vi "Read from File.vi"(7 "Section Name":string, 8 "error in (no error)":errorcluster, 10 "INI Ref":T1, 11 "Window Action in":refnum<class "Window Action.lvclass">) -> (0 "error out":errorcluster, 2 "INI Ref out":T1, 3 "Window Action out":refnum<class "Window Action.lvclass">)   [LabVIEW 2020, in "MacroAssert.lvlib" / "Window Action.lvclass"]
doc: "Reads associated parameters from the file identified by <B>INI Ref</B>."
uses:
  Window Action.lvclass
  <vilib>/Utility/config.llb/Config Data RefNum.ctl
  Window Action Type.ctl
  <vilib>/Utility/error.llb/Error Cluster From Error Code.vi
  <vilib>/Utility/config.llb/Read Key (String).vi
  Action Step/Action Step.lvclass
  MacroAssert.lvlib
  <vilib>/Utility/config.llb/NI_LVConfig.lvlib
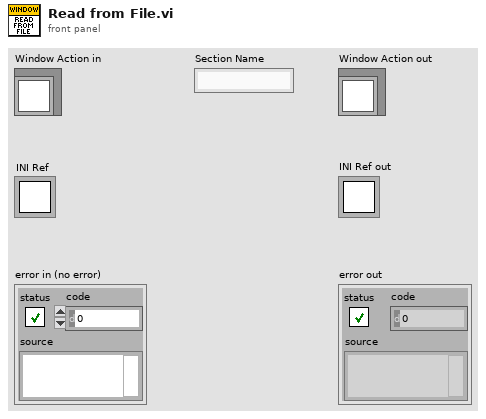
[diagram p1: front panel]
types:
  T1 = typedef "NI_LVConfig.lvlib/Config Data RefNum.ctl" = refnum<k1>
  T2 = typedef "MacroAssert.lvlib/Window Action.lvclass/Window Action Type.ctl" = enum16{"Maximize Window", "Restore Window", "Minimize Window", "Close Window", "Bring Window to Front", "Send Window to Back"}
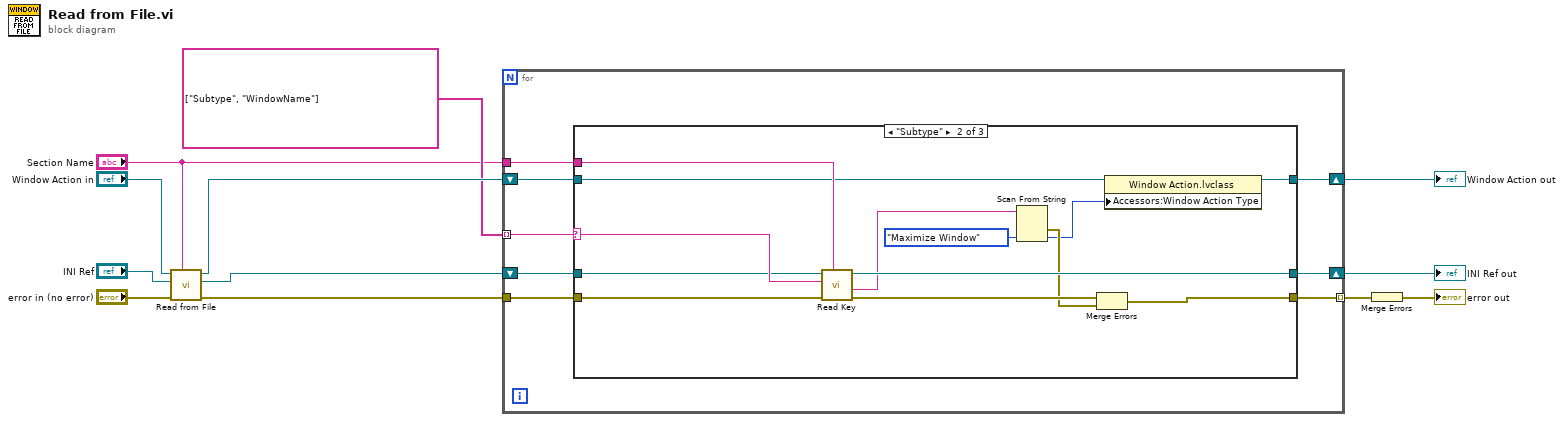
[diagram p0: block diagram]
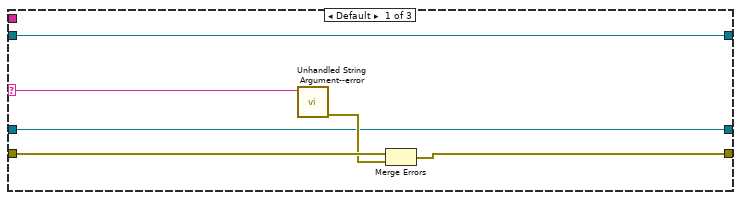
[diagram p2: hidden frame]
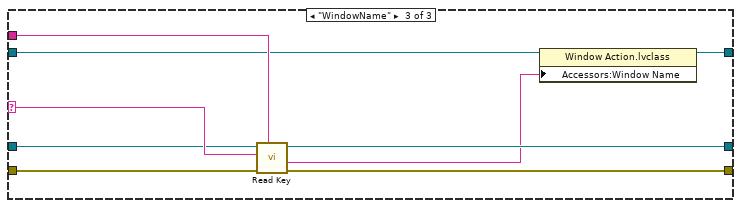
[diagram p3: hidden frame]
diagram:
  n1 = call-parent "Read from File.vi"("Section Name"="Section Name", "error in (no error)"="error in (no error)", "INI Ref"="INI Ref", "Step in"="Window Action in") -> ("error out"=w10:errorcluster, "INI Ref out"=w9:T1, "Step out"=w12:refnum<class "Window Action.lvclass">)  [unwired: 5 in]
  n2 = for {
    tunnel: string[] ["Subtype", "WindowName"] -> [w20] mode=indexing
    tunnel: w10 -> [w19]
    tunnel: "Section Name" -> [w18]
    shift-right: [w16] -> w2
    shift-left: w12 -> [w17]
    tunnel: [w15] -> w8 mode=indexing
    shift-right: [w13] -> w3
    shift-left: w9 -> [w14]
    n3 = case shown="\"Subtype\"" w20 {
      selector: w20 -> [w23 w34 w43]
      tunnel: w19 -> [w25 w39 w48]
      tunnel: w18 -> [_ w38 w47]
      tunnel: w17 -> [w26 w37 w46]
      tunnel: [w26 w36 w45] -> w16
      tunnel: [w22 w30 w44] -> w15
      tunnel: w14 -> [w21 w33 w42]
      tunnel: [w21 w32 w41] -> w13
      frame Default {
        n4 = call "Unhandled String Argument--error.vi"("Argument"=w23) -> ("error out"=w24:errorcluster)  [unwired: 10 in]
        n5 = Merge Errors(w25, w24) -> (w22:errorcluster)
      }
      frame "Subtype" {
        n6 = call-poly <vilib>:"Read Key.vi"("section"=w38, "error in (no error)"=w39, "key"=w34, "refnum"=w33) -> ("error out"=w35:errorcluster, "value"=w31:string, "refnum out"=w32:T1)  [unwired: 4 in, 1 out]
        n7 = Scan From String(input string=w31, default 1=Window_Action_Type."Maximize Window" ("Window Action Type")) -> (error out=w29:errorcluster, output 1=w28:T2)  [unwired: 3 in, 2 out]
        n8 = Merge Errors(w35, w29) -> (w30:errorcluster)
        n9 = property class="Window Action.lvclass"(reference=w37, "Accessors:Window Action Type"=w28) -> (reference out=w36:refnum<class "Window Action.lvclass">)  [unwired: 1 in, 1 out]
      }
      frame "WindowName" {
        n10 = call-poly <vilib>:"Read Key.vi"("section"=w47, "error in (no error)"=w48, "key"=w43, "refnum"=w42) -> ("error out"=w44:errorcluster, "value"=w40:string, "refnum out"=w41:T1)  [unwired: 4 in, 1 out]
        n11 = property class="Window Action.lvclass"(reference=w46, "Accessors:Window Name"=w40) -> (reference out=w45:refnum<class "Window Action.lvclass">)  [unwired: 1 in, 1 out]
      }
    }
  }
  "Window Action out" <- w2
  "INI Ref out" <- w3
  n12 = Merge Errors(w8) -> (→"error out":errorcluster)
